vi "Obtain Broadcast Events.vi"(8 "error in (no error)":errorcluster, 10 "Create New? (F)":bool) -> (0 "error out":errorcluster, 2 "Acquisition Broadcast Events":T1)   [LabVIEW 2019, in "Acquisition.lvlib"]
doc: "This VI Obtains/Creates the Broadcast events that will be used for other modules to register to receive messages from the module that owns this VI.\n\n<b>NOTE</b>: The contents of this VI are automatically generated and modified by the <b>Tools > Delacor > DQMH</b> utilities. Consider using those utilities instead of making your own modifications to this VI.\n_____\nBased on Delacor QMH Project Template 4.0.0.47.\n_____\nBased on Delacor QMH Project Template 5.0.0.82."
uses:
  Acquisition.lvlib
  Broadcast Events--cluster.ctl
  Did Init Argument--cluster.ctl
  Status Updated Argument--cluster.ctl
  Error Reported Argument--cluster.ctl
  Stop Argument--cluster.ctl
  Get Module Execution Status Argument--cluster.ctl
  Acquisition Started Argument--cluster.ctl
  Acquisition Stopped Argument--cluster.ctl
  Data Updated Argument--cluster.ctl
  Device Calibrated Argument--cluster.ctl
panel:
  # "NOTE: The contents of this VI are automatically generated and modified by the Tools > Delacor > DQMH utilities. Consider using those utilities instead of making your own modifications to this VI."
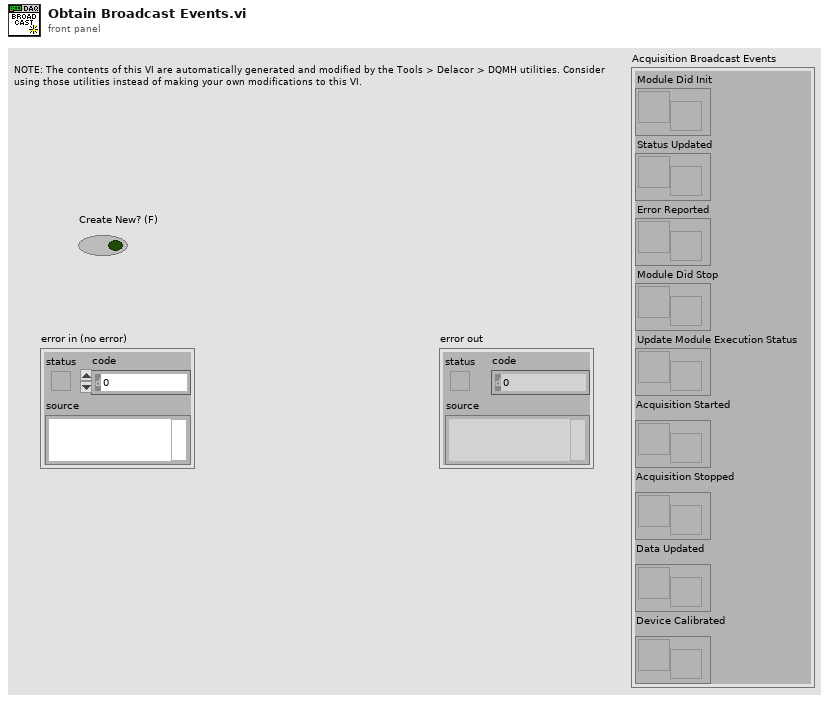
[diagram p1: front panel]
types:
  T1 = typedef "Acquisition.lvlib/Broadcast Events--cluster.ctl" = cluster{"Module Did Init":refnum<user-event>, "Status Updated":refnum<user-event>, "Error Reported":refnum<user-event>, "Module Did Stop":refnum<user-event>, "Update Module Execution Status":refnum<user-event>, "Acquisition Started":refnum<user-event>, "Acquisition Stopped":refnum<user-event>, "Data Updated":refnum<user-event>, "Device Calibrated":refnum<user-event>}
  T2 = typedef "Acquisition.lvlib/Device Calibrated Argument--cluster.ctl" = cluster{"Boolean":bool}
  T3 = typedef "Acquisition.lvlib/Data Updated Argument--cluster.ctl" = cluster{"Graph Data":waveform(dbl)[]}
  T4 = typedef "Acquisition.lvlib/Acquisition Stopped Argument--cluster.ctl" = cluster{"Boolean":bool}
  T5 = typedef "Acquisition.lvlib/Acquisition Started Argument--cluster.ctl" = cluster{"HW ID":string}
  T6 = typedef "Acquisition.lvlib/Get Module Execution Status Argument--cluster.ctl" = cluster{"Running?":bool}
  T7 = typedef "Acquisition.lvlib/Stop Argument--cluster.ctl" = cluster{"Origin":string, "Exit via Stop Module Req?":bool, "Wait for Module to stop?":bool}
  T8 = typedef "Acquisition.lvlib/Error Reported Argument--cluster.ctl" = cluster{"Error":errorcluster, "Additional Information":string, "Module Name":string}
  T9 = typedef "Acquisition.lvlib/Status Updated Argument--cluster.ctl" = cluster{"Status":string}
  T10 = typedef "Acquisition.lvlib/Did Init Argument--cluster.ctl" = cluster{"Init?":bool, "Info":string}
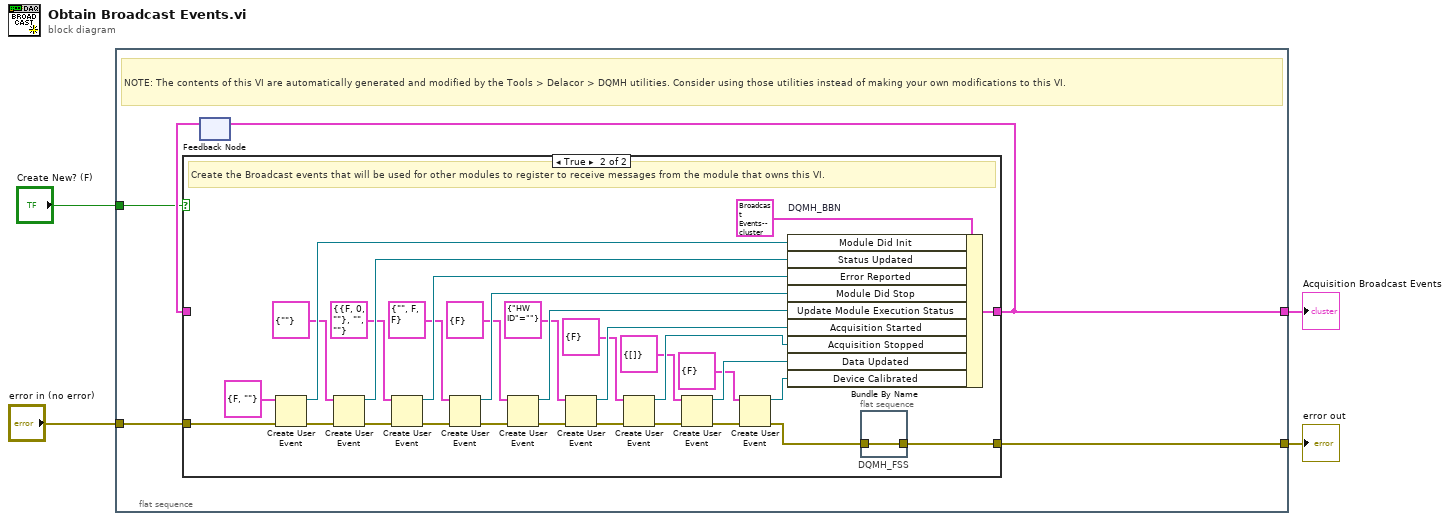
[diagram p0: block diagram]
diagram:
  n1 = flat-sequence {
    tunnel: [w9] -> w4
    tunnel: "error in (no error)" -> [w8]
    tunnel: [w6] -> w2
    tunnel: "Create New? (F)" -> [w5]
    frame #0 {
      # "NOTE: The contents of this VI are automatically generated and modified by the Tools > Delacor > DQMH utilities. Consider using those utilities instead of making your own modifications to this VI."
      n2 = feedback #1() -> (w7:T1)  [unwired: 1 in]
      n3 = case shown="True" w5 {
        tunnel: [w10 w27] -> w9
        tunnel: w8 -> [w10 w42]
        tunnel: [w11 w39] -> w6
        tunnel: w7 -> [w11 _]
        frame False {
          # "Obtain the Broadcast events that were created in a previous call to this VI."
        }
        frame True {
          # "Create the Broadcast events that will be used for other modules to register to receive messages from the module that owns this VI."
          n4 = Create User Event(user event datatype=T10 {"Init?"=FALSE, "Info"=""} ("Did Init Argument"), error in=w42) -> (user event=w40:refnum<user-event>, error out=w37:errorcluster)
          n5 = Create User Event(user event datatype=T9 {"Status"=""} ("Status Updated Argument"), error in=w37) -> (user event=w34:refnum<user-event>, error out=w36:errorcluster)
          n6 = Create User Event(user event datatype=T8 {"Error"={"status"=FALSE, "code"=0, "source"=""}, "Additional Information"="", "Module Name"=""} ("Error Reported Argument"), error in=w36) -> (user event=w31:refnum<user-event>, error out=w33:errorcluster)
          n7 = Create User Event(user event datatype=T7 {"Origin"="", "Exit via Stop Module Req?"=FALSE, "Wait for Module to stop?"=FALSE} ("Stop Argument"), error in=w33) -> (user event=w29:refnum<user-event>, error out=w28:errorcluster)
          n8 = Create User Event(user event datatype=T6 {"Running?"=FALSE} ("Get Module Execution Status Argument"), error in=w28) -> (user event=w25:refnum<user-event>, error out=w26:errorcluster)
          n9 = Create User Event(user event datatype=T5 {"HW ID"=""} ("Acquisition Started Argument"), error in=w26) -> (user event=w22:refnum<user-event>, error out=w23:errorcluster)
          n10 = Create User Event(user event datatype=T4 {"Boolean"=FALSE} ("Acquisition Stopped Argument"), error in=w23) -> (user event=w19:refnum<user-event>, error out=w20:errorcluster)
          n11 = Create User Event(user event datatype=T3 {"Graph Data"=[]} ("Data Updated Argument"), error in=w20) -> (user event=w16:refnum<user-event>, error out=w17:errorcluster)
          n12 = Create User Event(user event datatype=T2 {"Boolean"=FALSE} ("Device Calibrated Argument"), error in=w17) -> (user event=w13:refnum<user-event>, error out=w14:errorcluster)
          n13 = Bundle By Name "DQMH_BBN"(cluster=T1 {"Module Did Init"=refnum, "Status Updated"=refnum, "Error Reported"=refnum, "Module Did Stop"=refnum, "Update Module Execution Status"=refnum, "Acquisition Started"=refnum, "Acquisition Stopped"=refnum, "Data Updated"=refnum, "Device Calibrated"=refnum} ("output cluster"), "Module Did Init"=w40, "Status Updated"=w34, "Error Reported"=w31, "Module Did Stop"=w29, "Update Module Execution Status"=w25, "Acquisition Started"=w22, "Acquisition Stopped"=w19, "Data Updated"=w16, "Device Calibrated"=w13) -> (w39:T1)
          n14 = flat-sequence "DQMH_FSS" {
            tunnel: w14 -> [w43]
            tunnel: [w43] -> w27
            frame #0 {
            }
          }
        }
      }
      n15 = feedback-in #1(w6) -> ()
    }
  }
  "Acquisition Broadcast Events" <- w2
  "error out" <- w4
